vi "cm_Set Level Meter Colors.vi"(7 "Action":T1(ring), 8 "error in":errorcluster, 9 "Peak":u32, 10 "Current":u32, 11 "Channel Status":refnum<vi>) -> (0 "error out":errorcluster)   [LabVIEW 2012, in "Channel Monitor.xctl"]
uses:
  Channel Monitor.xctl
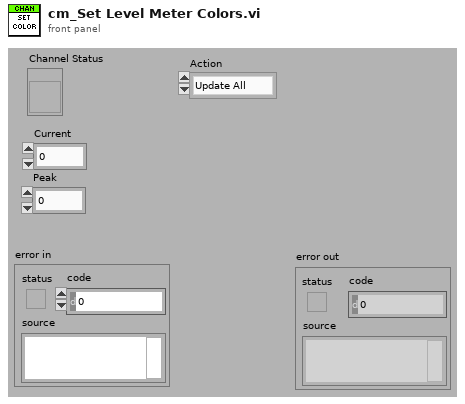
[diagram p1: front panel]
types:
  T1 = enum16{"Update All", "Current Only", "Peak Only"}
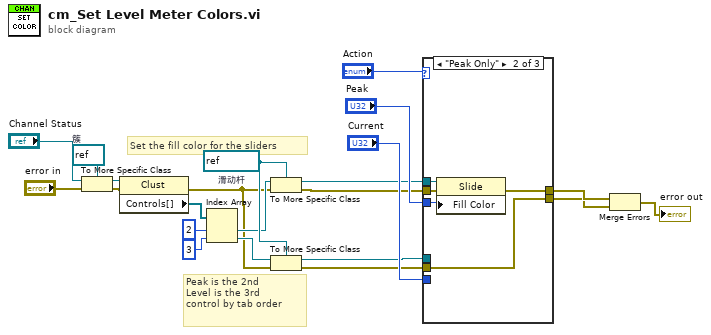
[diagram p0: block diagram]
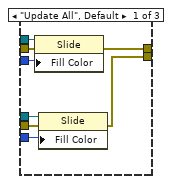
[diagram p2: hidden frame]
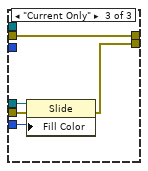
[diagram p3: hidden frame]
diagram:
  w18 = refnum<vi> refnum  # 滑动杆
  w10 = refnum<vi> refnum  # 簇
  # "Set the fill color for the sliders"
  # "Peak is the 2nd\nLevel is the 3rd\ncontrol by tab order"
  n1 = To More Specific Class(target class=w10, reference="Channel Status", error in="error in") -> (specific class reference=w7:refnum<vi>, error out=w14:errorcluster)
  n2 = property class="Clust"(reference=w7, error in=w14) -> (error out=w5:errorcluster, "Controls[]"=w8:refnum<vi>[])  [unwired: 1 out]
  n3 = Index Array(array=w8, index #1=2 ("index"), index #2=3 ("index")) -> (element #1=w9:refnum<vi>, element #2=w17:refnum<vi>)
  n4 = To More Specific Class(target class=w18, reference=w9, error in=w5) -> (specific class reference=w11:refnum<vi>, error out=w15:errorcluster)
  n5 = To More Specific Class(target class=w18, reference=w17, error in=w5) -> (specific class reference=w19:refnum<vi>, error out=w20:errorcluster)
  n6 = case shown="\"Peak Only\"" "Action" {
    tunnel: "Current" -> [w30 _ w40]
    tunnel: "Peak" -> [w29 w35 _]
    tunnel: w20 -> [w28 w31 w39]
    tunnel: w19 -> [w27 _ w38]
    tunnel: w15 -> [w26 w34 w36]
    tunnel: w11 -> [w25 w33 _]
    tunnel: [w24 w32 w36] -> w4
    tunnel: [w23 w31 w37] -> w3
    frame "Update All", Default {
      n7 = property class="Slide"(reference=w25, error in=w26, "Fill Color"=w29) -> (error out=w24:errorcluster)  [unwired: 1 out]
      n8 = property class="Slide"(reference=w27, error in=w28, "Fill Color"=w30) -> (error out=w23:errorcluster)  [unwired: 1 out]
    }
    frame "Peak Only" {
      n9 = property class="Slide"(reference=w33, error in=w34, "Fill Color"=w35) -> (error out=w32:errorcluster)  [unwired: 1 out]
    }
    frame "Current Only" {
      n10 = property class="Slide"(reference=w38, error in=w39, "Fill Color"=w40) -> (error out=w37:errorcluster)  [unwired: 1 out]
    }
  }
  n11 = Merge Errors(w4, w3) -> (→"error out":errorcluster)
